vi "ain_dio.vi"() -> ()   [LabVIEW 2019]
panel:
  in  "D6 Output":bool
  out "D6":bool
  out "D5":bool
  out "D4":bool
  out "D3":bool
  out "D2":bool
  out "D1":bool
  out "D0":bool
  in  "SampleRate":dbl=1000.0
  in  "DeviceDriver":string="DI320NT.DLL"
  out "Waveform Chart":dbl[](graph)
  out "Channel 1":dbl(knob) scale=-10.0..10.0
  in  "DataqSdk":refnum<k7>(container)
  in  "Start/Stop":bool
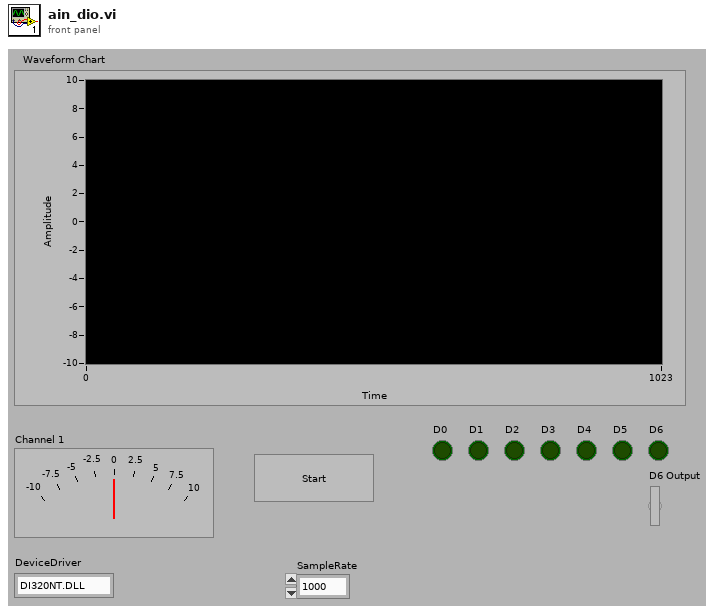
[diagram p1: front panel]
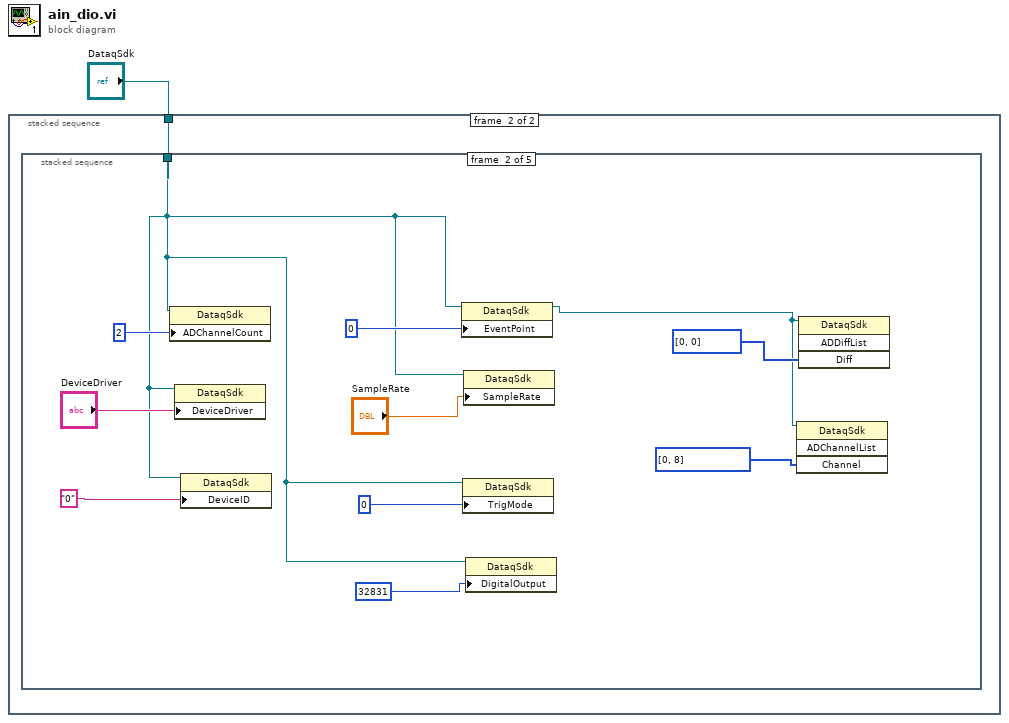
[diagram p0: block diagram]
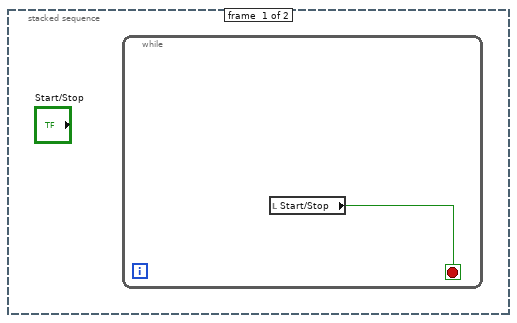
[diagram p2: hidden frame]
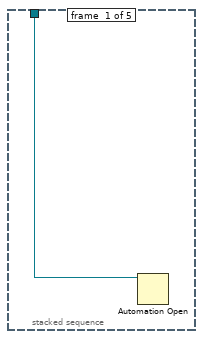
[diagram p3: hidden frame]
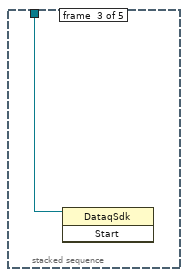
[diagram p4: hidden frame]
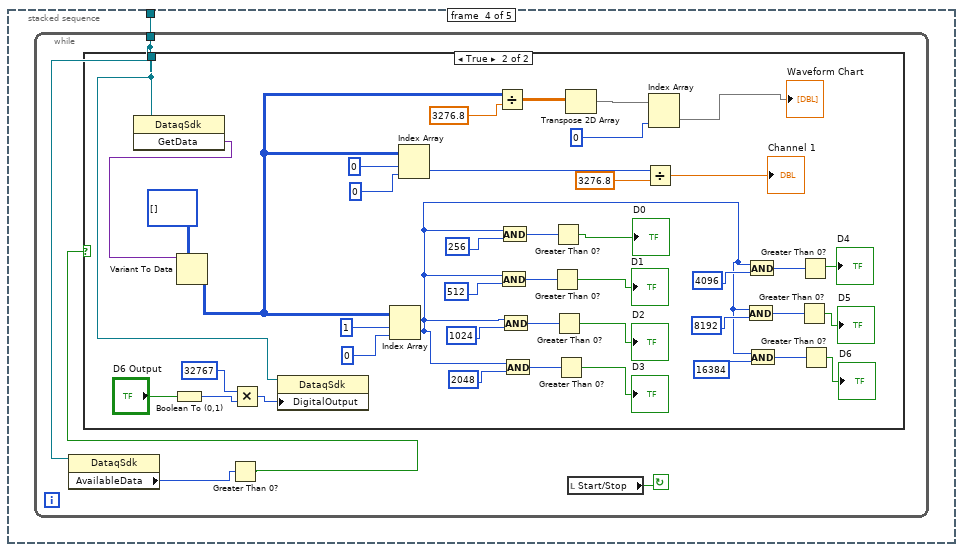
[diagram p5: hidden frame]
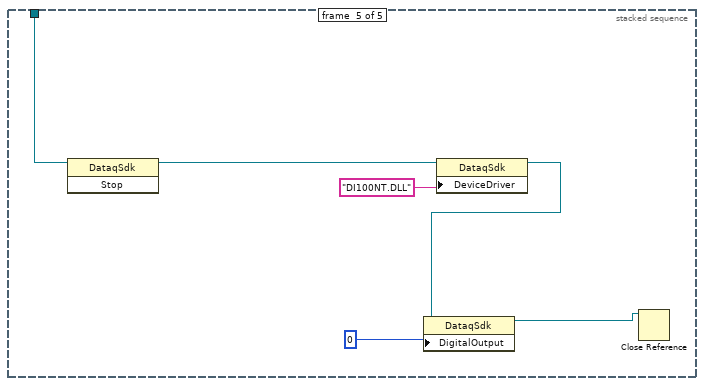
[diagram p7: hidden frame]
diagram:
  n1 = stacked-sequence {
    tunnel: "DataqSdk" -> [_ w3]
    frame #0 {
      n2 = while {
        stop <- w2 stop-if-true
        n3 = local read "Start/Stop"() -> (w2:bool)
      }
    }
    frame #1 {
      n4 = stacked-sequence {
        tunnel: w3 -> [w4 w6 w16 w17 w69]
        frame #0 {
          n5 = Automation Open(Automation Refnum=w4) -> ()  [unwired: 3 in, 2 out]
        }
        frame #1 {
          n6 = property class="DataqSdk"(reference=w6, "ADChannelCount"=2) -> ()  [unwired: 1 in, 2 out]
          n7 = property class="DataqSdk"(reference=w6, "DeviceDriver"="DeviceDriver") -> ()  [unwired: 1 in, 2 out]
          n8 = property class="DataqSdk"(reference=w6, "DeviceID"="0") -> ()  [unwired: 1 in, 2 out]
          n9 = property class="DataqSdk"(reference=w6, "EventPoint"=0) -> (reference out=w7:refnum<k7>)  [unwired: 1 in, 1 out]
          n10 = property class="DataqSdk"(reference=w6, "TrigMode"=0) -> ()  [unwired: 1 in, 2 out]
          n11 = property class="DataqSdk"(reference=w6, "SampleRate"="SampleRate") -> ()  [unwired: 1 in, 2 out]
          n12 = property class="DataqSdk"(reference=w6, "DigitalOutput"=u16 32831) -> ()  [unwired: 1 in, 2 out]
          n13 = invoke class="DataqSdk" method="ADChannelList"(reference=w7, "Channel"=i32[] [0, 8] ("Array")) -> ()  [unwired: 2 in, 4 out]
          n14 = invoke class="DataqSdk" method="ADDiffList"(reference=w7, "Diff"=i32[] [0, 0] ("Array")) -> ()  [unwired: 2 in, 4 out]
        }
        frame #2 {
          n15 = invoke class="DataqSdk" method="Start"(reference=w16) -> ()  [unwired: 2 in, 3 out]
        }
        frame #3 {
          n16 = while {
            tunnel: w17 -> [w20]
            stop <- w21 continue-if-true
            n17 = property class="DataqSdk"(reference=w20) -> ("AvailableData"=w19:i32)  [unwired: 1 in, 2 out]
            n18 = Greater Than 0?(x=w19) -> (x > 0?=w18:bool)
            n19 = case shown="True" w18 {
              tunnel: w20 -> [_ w26]
              frame False {
              }
              frame True {
                n20 = invoke class="DataqSdk" method="GetData"(reference=w26) -> ("GetData"=w60:variant)  [unwired: 2 in, 2 out]
                n21 = Boolean To (0,1)(Boolean="D6 Output") -> (0, 1=w23:i16)
                n22 = Variant To Data(type=i16[][] [], Variant=w60) -> (data=w54:i16[][])  [unwired: 1 in, 1 out]
                n23 = Multiply(x=32767, y=w23) -> (x*y=w22:i32)
                n24 = property class="DataqSdk"(reference=w26, "DigitalOutput"=w22) -> ()  [unwired: 1 in, 2 out]
                n25 = Index Array(array=w54, index (row)=1, index (col)=0) -> (element=w34:i16)
                n26 = Index Array(array=w54, index (row)=0, index (col)=0) -> (element=w53:i16)
                n27 = Divide(x=w54, y=3276.8) -> (x/y=w30:dbl[][])
                n28 = And(x=w34, y=512) -> (x .and. y?=w48:i32)
                n29 = And(x=w34, y=256) -> (x .and. y?=w51:i32)
                n30 = And(x=w34, y=1024) -> (x .and. y?=w46:i32)
                n31 = And(x=w34, y=2048) -> (x .and. y?=w44:i32)
                n32 = Greater Than 0?(x=w48) -> (x > 0?=→"D1":bool)
                n33 = Greater Than 0?(x=w51) -> (x > 0?=→"D0":bool)
                n34 = Greater Than 0?(x=w46) -> (x > 0?=→"D2":bool)
                n35 = Greater Than 0?(x=w44) -> (x > 0?=→"D3":bool)
                n36 = Transpose 2D Array(2D array=w30) -> (transposed array=w29:dbl[][])
                n37 = Divide(x=w53, y=3276.8) -> (x/y=→"Channel 1":dbl)
                n38 = Index Array(array=w29, index (col)=0) -> (element=→"Waveform Chart":dbl[])  [unwired: 1 in]
                n39 = And(x=w34, y=8192) -> (x .and. y?=w37:i32)
                n40 = And(x=w34, y=4096) -> (x .and. y?=w39:i32)
                n41 = And(x=w34, y=16384) -> (x .and. y?=w35:i32)
                n42 = Greater Than 0?(x=w37) -> (x > 0?=→"D5":bool)
                n43 = Greater Than 0?(x=w39) -> (x > 0?=→"D4":bool)
                n44 = Greater Than 0?(x=w35) -> (x > 0?=→"D6":bool)
              }
            }
            n45 = local read "Start/Stop"() -> (w21:bool)
          }
        }
        frame #4 {
          n46 = invoke class="DataqSdk" method="Stop"(reference=w69) -> (reference out=w65:refnum<k7>)  [unwired: 2 in, 2 out]
          n47 = property class="DataqSdk"(reference=w65, "DeviceDriver"="DI100NT.DLL") -> (reference out=w68:refnum<k7>)  [unwired: 1 in, 1 out]
          n48 = property class="DataqSdk"(reference=w68, "DigitalOutput"=0) -> (reference out=w64:refnum<k7>)  [unwired: 1 in, 1 out]
          n49 = Close Reference(reference=w64) -> ()  [unwired: 1 in, 1 out]
        }
      }
    }
  }
